vi "BalanceMotorControl.vi"() -> ()   [LabVIEW 2017]
uses:
  <vilib>/addons/control/pid/pid.llb/PID (DBL Array).vi
  <vilib>/addons/control/pid/NI_PID_pid.lvlib
panel:
  out "Gx,Gy, OmegaZ":dbl[](array[numeric])
  in  "Number of Motors":i16
  in  "PID gains":T1(array[cluster]) {"derivative time (Td, min)" format="%.3f"; "integral time (Ti, min)" format="%.3f"; "proportional gain (Kc)" format="%.3f"}
  in  "Alpha, Beta, Gamma":dbl[](array[numeric])
  # "The inputs for this vi are errors from the desired orientation (angles) and the outputs are corrections in the percent power for the 6 motors."
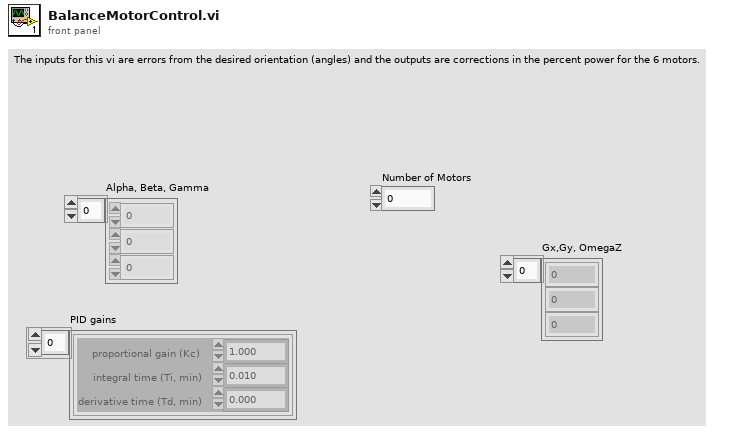
[diagram p1: front panel]
types:
  T1 = cluster{"proportional gain (Kc)":dbl, "integral time (Ti, min)":dbl, "derivative time (Td, min)":dbl}[]
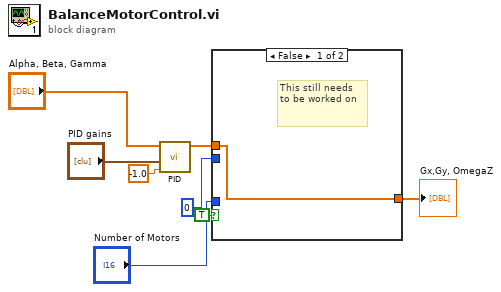
[diagram p0: block diagram]
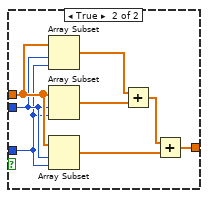
[diagram p2: hidden frame]
diagram:
  n1 = call-poly <vilib>:"PID.vi"("dt (s)"=-1.0, "PID gains"="PID gains", "setpoint"="Alpha, Beta, Gamma") -> ("output"=w5:dbl[])  [unwired: 7 in, 1 out]
  n2 = case shown="False" TRUE {
    tunnel: w5 -> [w9 w17]
    tunnel: "Number of Motors" -> [_ w15]
    tunnel: 0 ("index") -> [_ w16]
    tunnel: [w9 w10] -> w2
    frame False {
      # "This still needs \nto be worked on"
    }
    frame True {
      n3 = Array Subset "Array Subset"(array=w17, index=w16, length=w15) -> (w14:dbl[])
      n4 = Array Subset(array=w17, index=w16, length=w15) -> (w13:dbl[])
      n5 = Array Subset(array=w17, index=w16, length=w15) -> (w12:dbl[])
      n6 = Add(x=w14, y=w13) -> (x+y=w11:dbl[])
      n7 = Add(x=w11, y=w12) -> (x+y=w10:dbl[])
    }
  }
  "Gx,Gy, OmegaZ" <- w2
